vi "Log Error.vi"(4 "Context":string="(unknown)", 6 "Facility (default)":T1="default", 8 "error in (no error)":errorcluster) -> (0 "error out":errorcluster)   [LabVIEW 2017, in "Log.lvclass"]
uses:
  Log.lvclass
  Log_Facilities.ctl
  Log_Facility.ctl
  Log_Level.ctl
  <vilib>/Utility/error.llb/DialogType.ctl
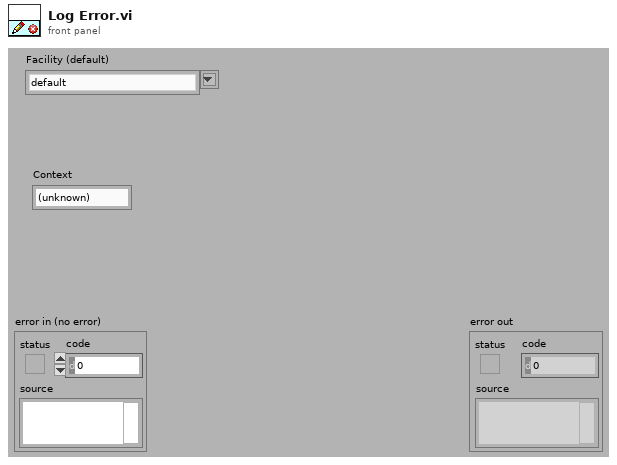
[diagram p1: front panel]
types:
  T1 = typedef "Log.lvclass/Log_Facilities.ctl" = string
  T2 = typedef "Log.lvclass/Log_Facility.ctl" = cluster{"Path":path, "Ref":refnum<file>, "Level":T3}
  T3 = typedef "Log.lvclass/Log_Level.ctl" = enum16{"none", "info", "trace", "warn", "error", "fatal"}
  T4 = typedef "DialogType.ctl" = u16
  T5 = typedef "Log.lvclass/ObjectAttributes.ctl" = cluster{"Level":T3, "Facilities":variant, "Event":refnum<user-event>}
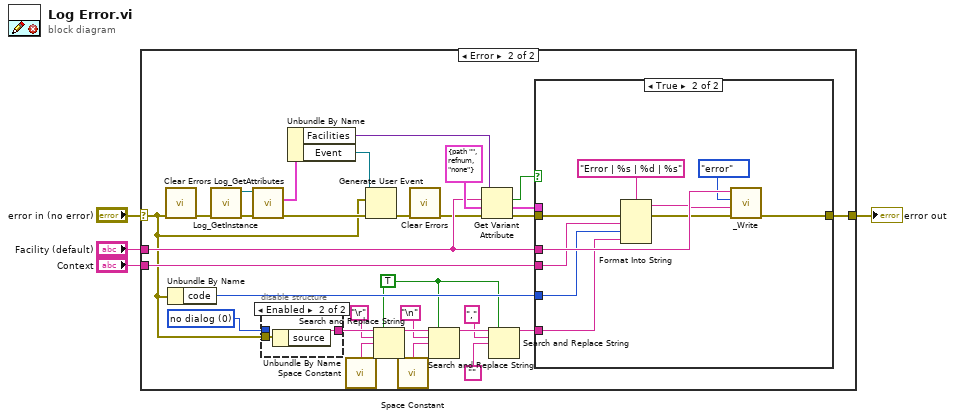
[diagram p0: block diagram]
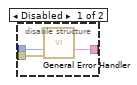
[diagram p3: hidden frame]
diagram:
  n1 = case shown="Error" "error in (no error)" {
    selector: "error in (no error)" -> [w5 w12]
    tunnel: "Context" -> [_ w35]
    tunnel: [w5 w24] -> w3
    tunnel: "Facility (default)" -> [_ w23]
    frame No Error {
    }
    frame Error {
      w7 = TRUE
      w21 = T4 0 items=["no dialog", "OK message", "continue or stop message", "OK message + warnings", "continue/stop + warnings"] ("type of dialog (OK msg:1)")
      n2 = call <vilib>:"Clear Errors.vi"("error in (no error)"=w12) -> ("error out"=w25:errorcluster)  [unwired: 5 in, 1 out]
      n3 = Unbundle By Name(w12) -> ("code"=w22:i32)
      n4 = call "Log_GetInstance.vi"("error in (no error)"=w25) -> ("error out"=w34:errorcluster, "reference out"=w27:refnum<class "Log.lvclass">)  [unwired: 6 in, 3 out]
      n5 = call "Log_GetAttributes.vi"("error in (no error)"=w34, "reference in"=w27) -> ("error out"=w32:errorcluster, "Data"=w26:T5)  [unwired: 6 in, 2 out]
      n6 = disable-structure shown="Enabled" {
        disable-tunnel: w21 -> [w38 _]
        disable-tunnel: [w37 w39] -> w20
        disable-tunnel: w12 -> [w36 w40]
        frame Disabled {
          n7 = call <vilib>:"General Error Handler.vi"("type of dialog (OK msg:1)"=w38, "error in (no error)"=w36) -> ("message"=w37:string)  [unwired: 9 in, 4 out]
        }
        frame Enabled {
          n8 = Unbundle By Name(w40) -> ("source"=w39:string)
        }
      }
      n9 = Unbundle By Name(w26) -> ("Facilities"=w33:variant, "Event"=w13:refnum<user-event>)
      n10 = call <vilib>:"Space Constant.vi"() -> ("String"=w19:string)
      n11 = Generate User Event(user event=w13, event data cluster=w12, error in=w32) -> (error out=w14:errorcluster)  [unwired: 1 in, 1 out]
      n12 = Search and Replace String(replace all?=w7, input string=w20, search string="\r", replace string=w19) -> (result string=w17:string)  [unwired: 4 in, 3 out]
      n13 = call <vilib>:"Space Constant.vi"() -> ("String"=w15:string)
      n14 = call <vilib>:"Clear Errors.vi"("error in (no error)"=w14) -> ("error out"=w6:errorcluster)  [unwired: 5 in, 1 out]
      n15 = Search and Replace String(replace all?=w7, input string=w17, search string="\n", replace string=w15) -> (result string=w10:string)  [unwired: 4 in, 3 out]
      n16 = Get Variant Attribute(Variant=w33, name=w23, default value (empty Variant)=T2 {"Path"=path "", "Ref"=refnum, "Level"=enum."none"} ("Cluster"), error in=w6) -> (found=w28:bool, value=w30:T2, error out=w29:errorcluster)  [unwired: 1 out]
      n17 = Search and Replace String(replace all?=w7, input string=w10, search string="," ("format string"), replace string="") -> (result string=w9:string)  [unwired: 4 in, 3 out]
      n18 = case shown="True" w28 {
        tunnel: w30 -> [_ _]
        tunnel: w29 -> [w41 w51]
        tunnel: [w41 w50] -> w24
        tunnel: w23 -> [_ w49]
        tunnel: w35 -> [_ w46]
        tunnel: w22 -> [_ w43]
        tunnel: w9 -> [_ w42]
        frame False {
        }
        frame True {
          n19 = Format Into String(format string="Error | %s | %d | %s", error in=w51, w46, w43, w42) -> (resulting string=w45:string, error out=w47:errorcluster)  [unwired: 1 in]
          n20 = call "_Write.vi"("error in (no error)"=w47, "Message"=w45, "Level"=Log_Level."error", "Name"=w49) -> ("error out"=w50:errorcluster)  [unwired: 7 in]
        }
      }
    }
  }
  "error out" <- w3
